vi "Offset Locking- Main with Slave Tracking v2.1.vi"() -> ()   [LabVIEW 2018]
uses:
  <vilib>/Utility/error.llb/DialogType.ctl
  <vilib>/Analysis/1siggen.llb/Ramp Pattern by Samples.vi
  <vilib>/measure/mamon.llb/Waveform Peak Detection for 1 Chan.vi
  <vilib>/addons/control/pid/pid.llb/PID Advanced (DBL).vi
  <vilib>/measure/NI_MAPro.lvlib
  <vilib>/addons/control/pid/NI_PID_pid.lvlib
  <vilib>/Analysis/NI_AALBase.lvlib
  <vilib>/measure/NI_MABase.lvlib
panel:
  in  "width":i32=100
  in  "start":dbl format="%0.2f"
  in  "end":dbl=1.0 format="%0.2f"
  in  "samples":i32=128
  in  "Waveform Test?":bool
  in  "reset signal":bool
  in  "phase":dbl format="%.2p"
  out "Chirp Rate":dbl format="%#_g GHz/ms"
  out "Single Mode?":bool
  out "# of Peaks found when Chirping?":i32
  in  "Minimum amplitude for Slave":dbl=0.15 format="%.2p"
  in  "Minimum \namplitude\nfor peaks":dbl=0.8 format="%#_13g V"
  in  "PZT Voltage to \nFrequency Conversion":dbl=-1.41655 format="%#_g V/GHz"
  out "PZT Chirp Output":waveform(dbl)(graph)
  in  "offset":dbl format="%0.2p V"
  in  "Sampling Info":cluster{"Fs":dbl, "#s":dbl}={"Fs"=10000.0, "#s"=100.0} {"Fs" format="%.2p"}
  in  "frequency":dbl=10.0 format="%0.2p Hz"
  in  "Chirp Amplitude":dbl=1.5 format="%0.2p GHz"
  in  "Run Chirp Program?":bool
  out "Run Time (min)":dbl
  out "standard deviation":dbl format="%0.3e"
  in  "Ref Peak 2":i32=2
  in  "Ref Peak":i32=3
  in  "First Cal Peak":i32=2
  in  "Last Cal Peak":i32=4
  out "# found":i32
  out "Offset":dbl(graph)
  in  "Manual PZT Control":dbl format="%#_g V"
  in  "Engage PZT PID?":bool
  out "Offset (GHz)":dbl format="%#_4g"
  in  "# of Shots for Averaging":i32=100
  in  "Name Convention":string="Chirp Offset Lock Log"
  in  "Save Directory":path=path "C:/Users/LabUser/Google Drive/Measurements/04-2018"
  out "Four peaks?":bool
  out "PZT Output":dbl(graph)
  in  "PID Gains":T1={"proportional gain (Kc)"=-1.0, "integral time (Ti, min)"=0.01, "derivative time (Td, min)"=0.0} {"derivative time (Td, min)" format="%.3f"; "integral time (Ti, min)" format="%.3f"; "proportional gain (Kc)" format="%.3f"}
  in  "Setpoint Range (GHz)":cluster{"setpoint high":dbl, "setpoint low":dbl}={"setpoint high"=7.7901, "setpoint low"=7.7899} {"setpoint high" format="%.4f"; "setpoint low" format="%.4f"}
  out "dt out (s)":dbl format="%.3f"
  in  "Frequency Offset Setpoint (GHz)":dbl=7.79 format="%.3f"
  out "GHz/sec":dbl
  out "dt":dbl format="%#_4g"
  out "Locations":dbl[](array[numeric]) format="%.2p"
  out "Amplitudes":dbl[](array[numeric]) format="%.2p"
  out "2nd Derivatives":dbl[](array[numeric]) format="%.2p"
  out "10 GHz FPI":dynamicdata(graph)
  in  "Stop":bool
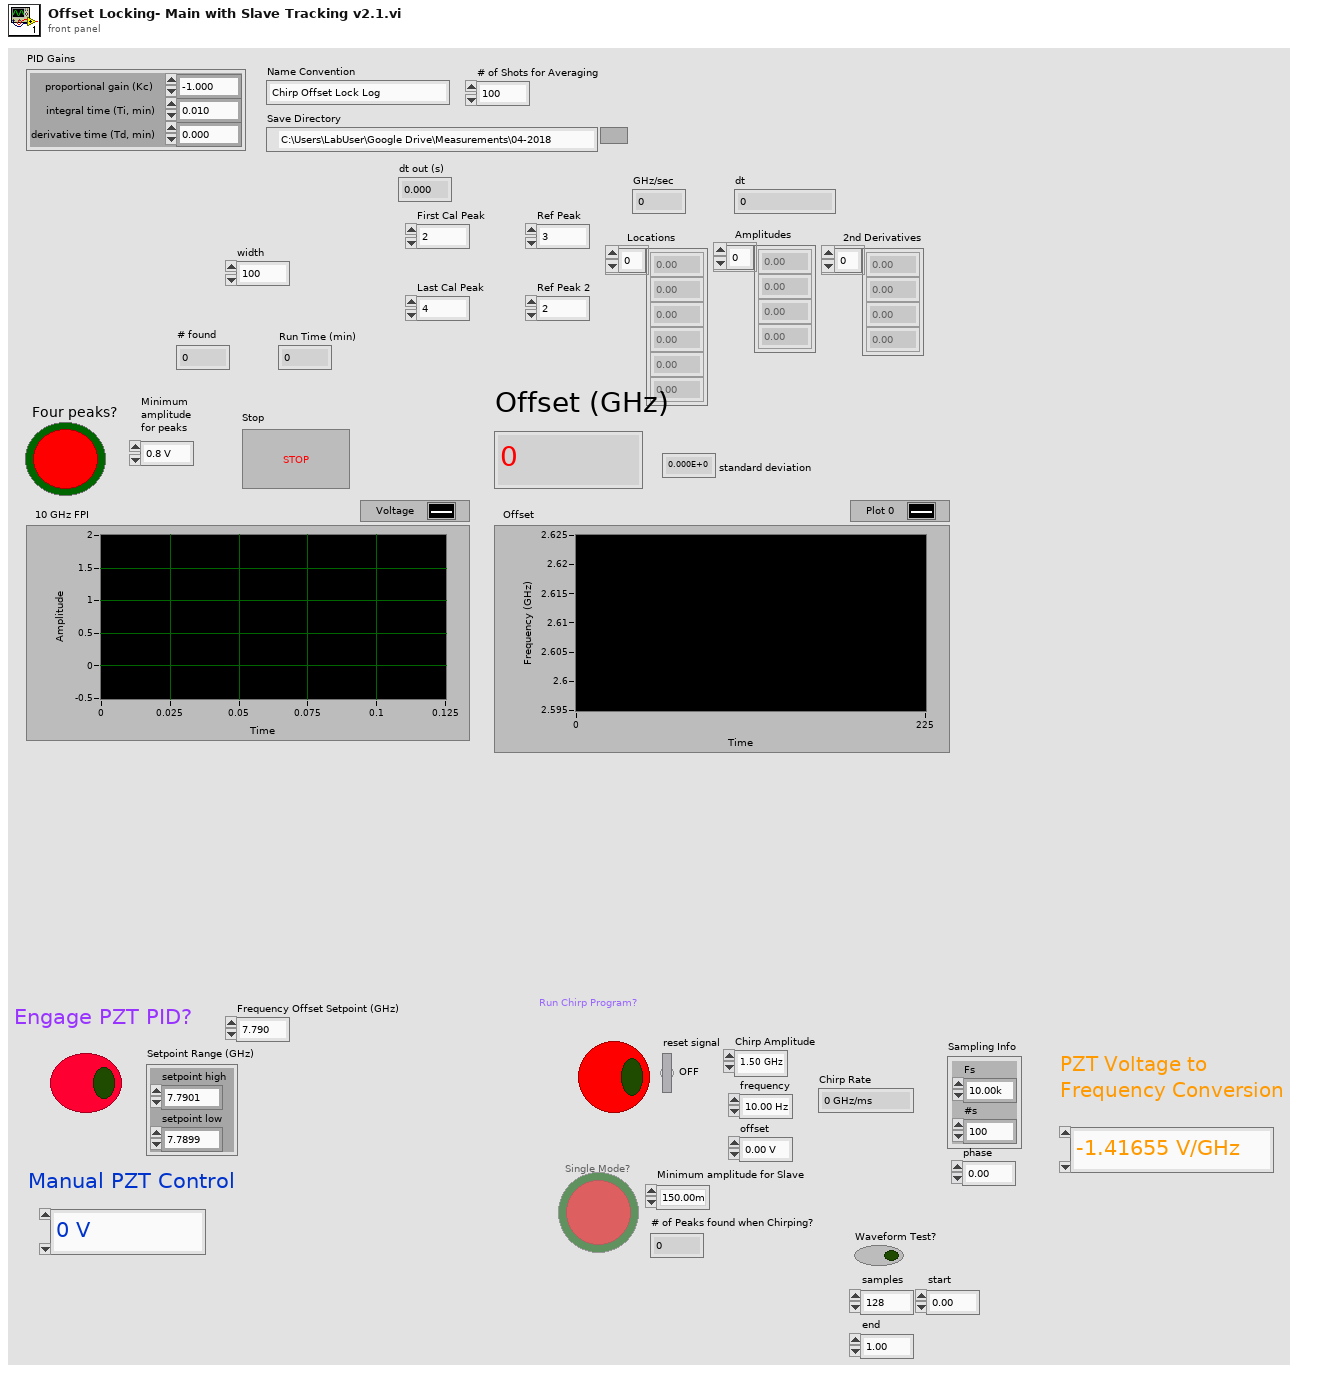
[diagram p1: front panel]
types:
  T1 = cluster{"proportional gain (Kc)":dbl, "integral time (Ti, min)":dbl, "derivative time (Td, min)":dbl}
  T2 = enum8{"Enabled", "Disabled", "Disabled and Grayed Out"}
  T3 = typedef "DialogType.ctl" = u16
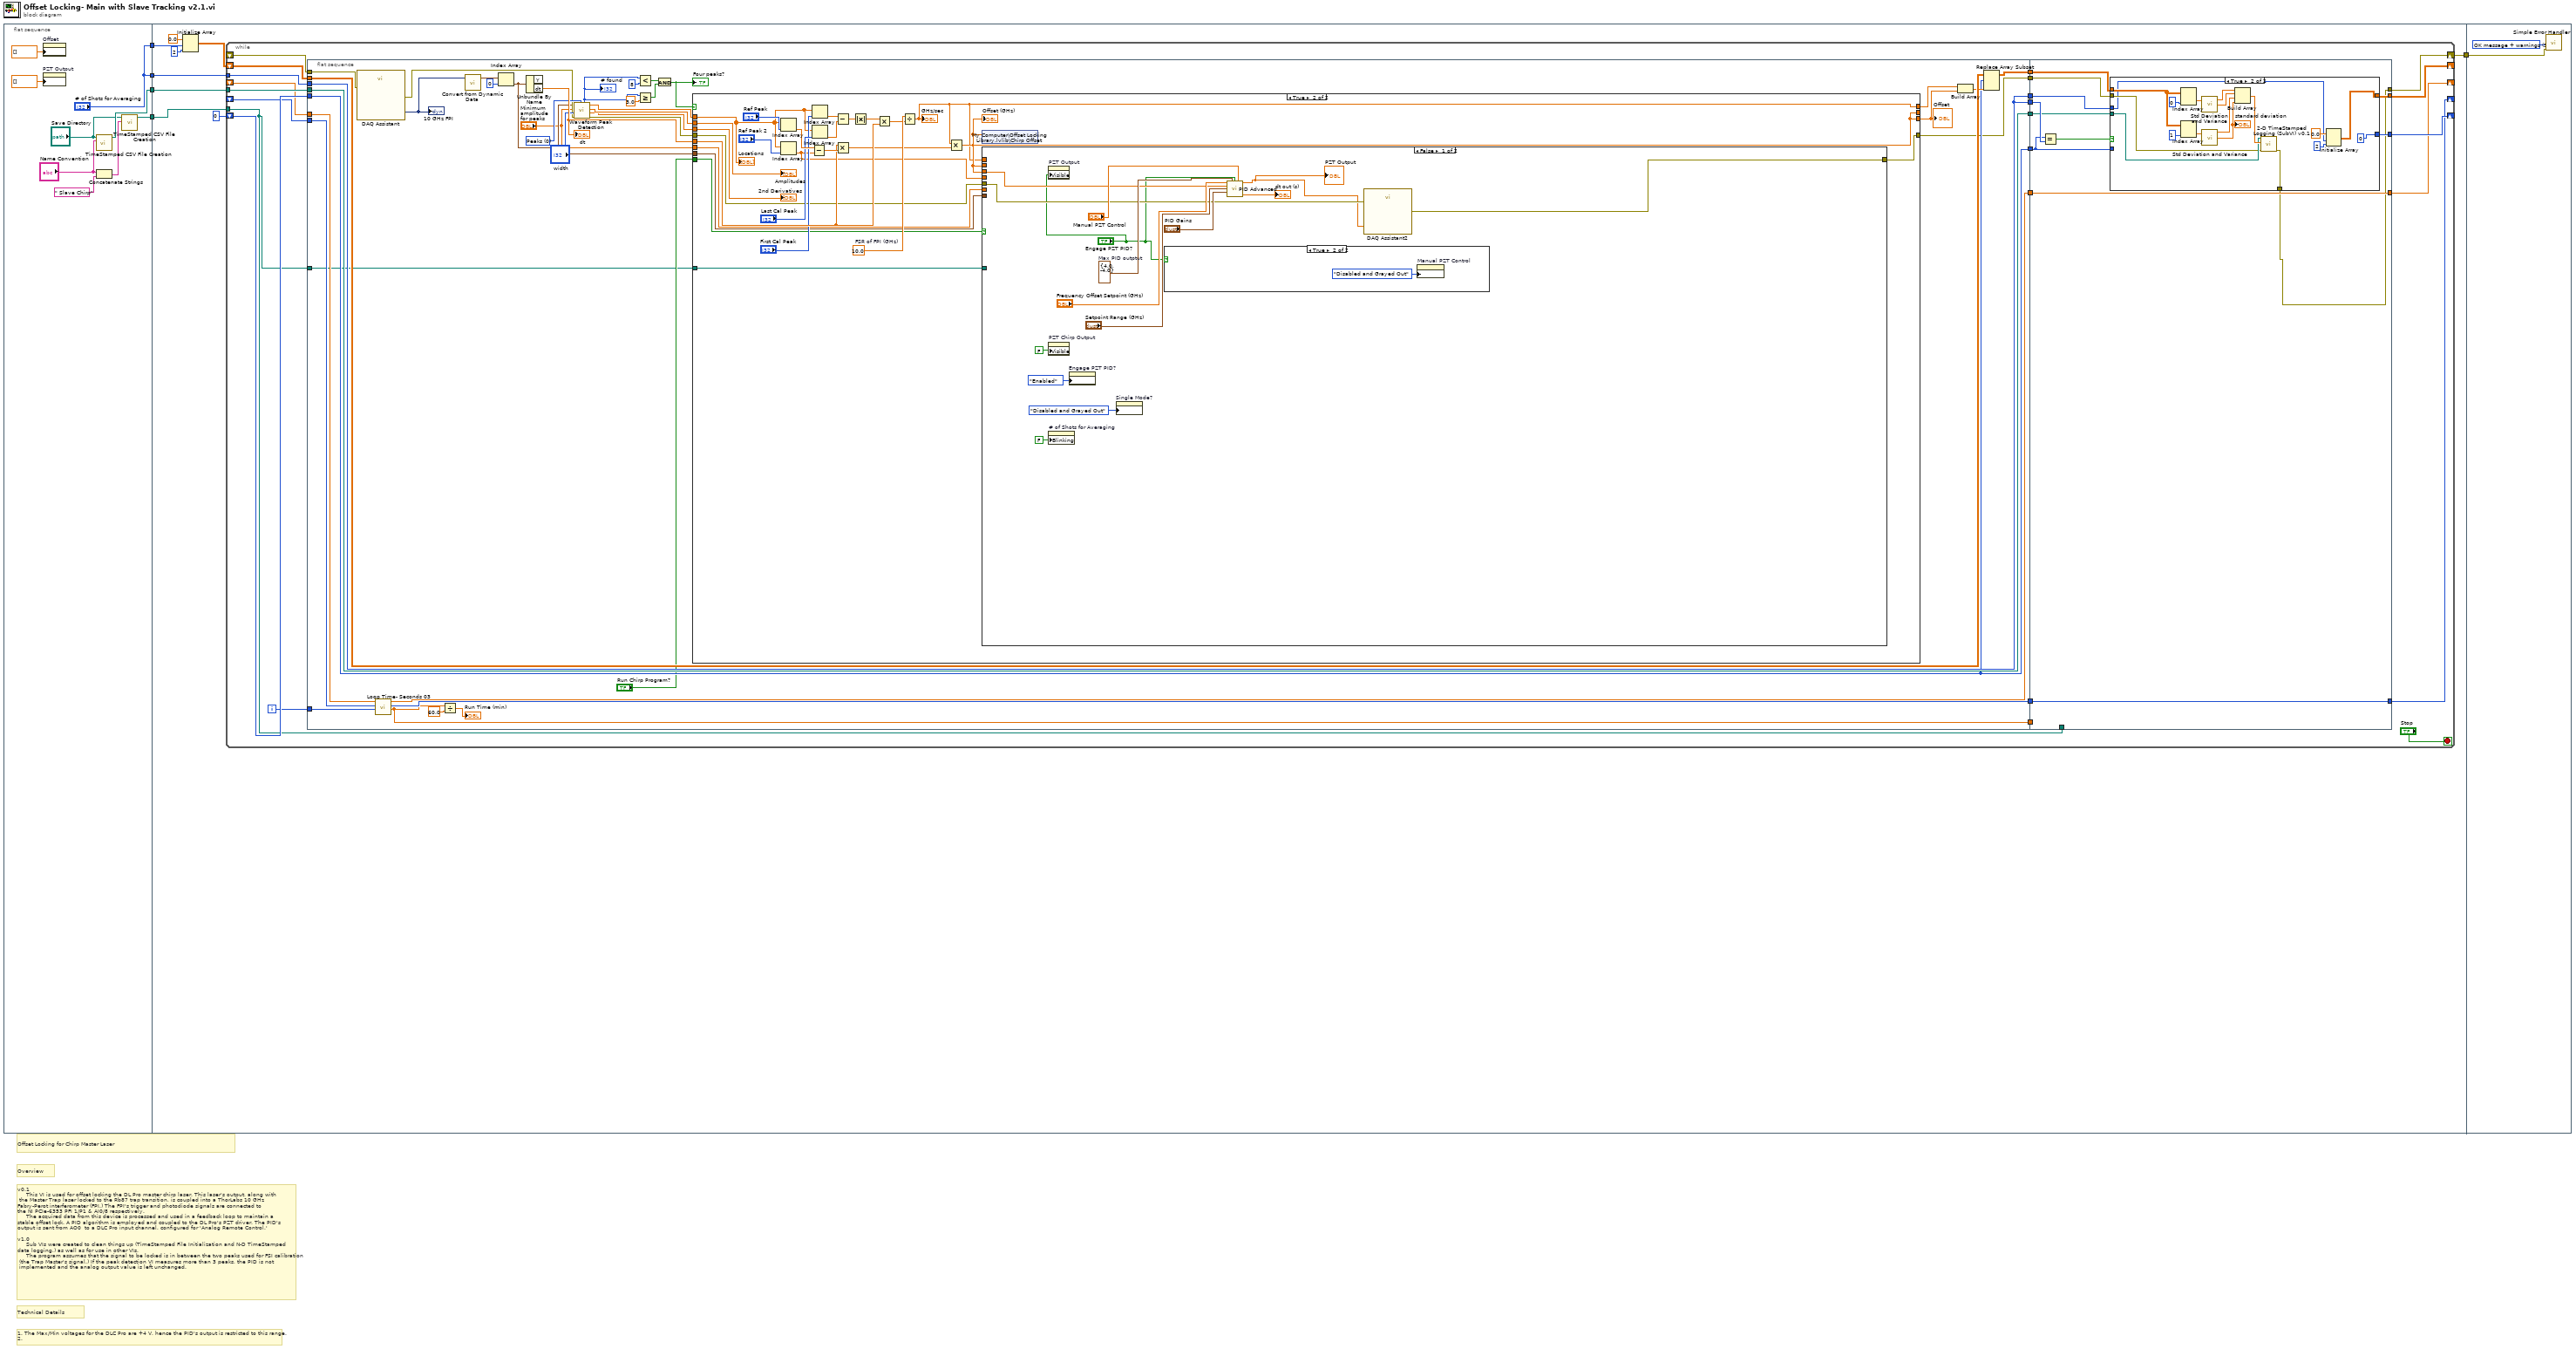
[diagram p0: block diagram]
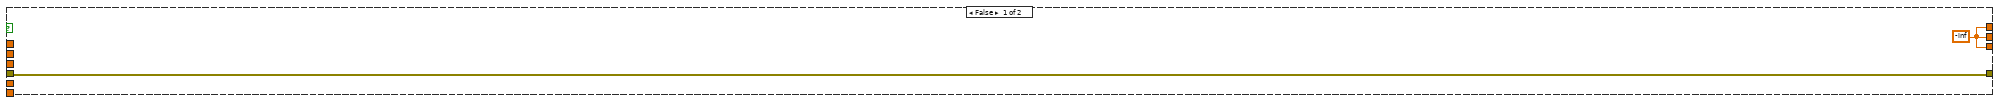
[diagram p2: hidden frame]
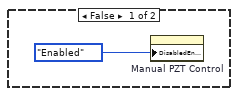
[diagram p3: hidden frame]
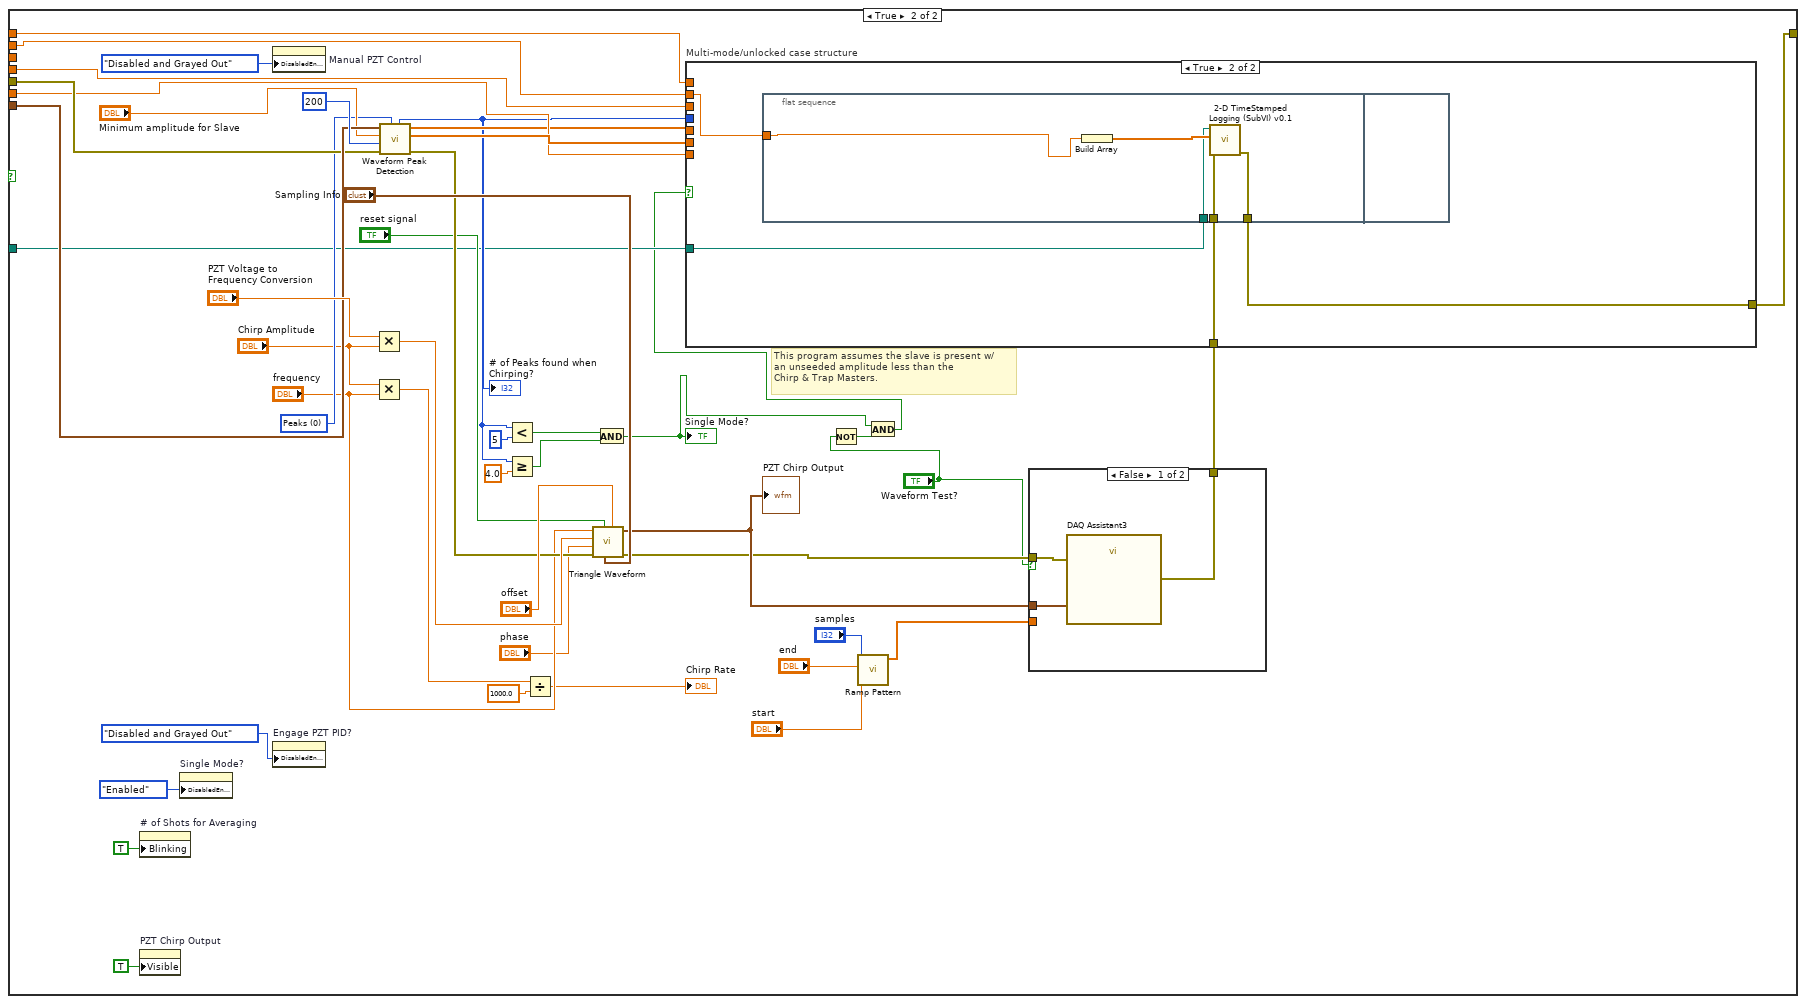
[diagram p4: hidden frame]
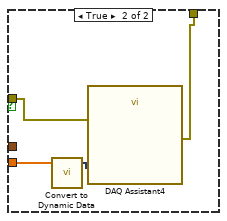
[diagram p5: hidden frame]
diagram:
  # "1. The Max/Min voltages for the DLC Pro are +4 V, hence the PID's output is restricted to this range.\n2."
  # "Technical Details"
  # "v0.1\n     This VI is used for offset locking the DL Pro master chirp laser. This laser's output, along with\n the Master Trap laser locked to the Rb87 trap transition, is coupled into a ThorLabs 10 GHz \nFabry-Perot interferometer (FPI.) The FPI's trigger and photodiode signals are connected to \nthe NI PCIe-6353 PFI 1/P1 & AI0/8 respectively. \n     The acquired data from this device is processed and used in a feedback loop to maintain a \nstable offset lock. A PID algorithm is employed and coupled to the DL Pro's PZT driver. The PID's\noutput is sent from AO0  to a DLC Pro input channel, configured for 'Analog Remote Control.'\n\nv1.0\n     Sub VIs were created to clean things up (TimeStamped File Initialization and N-D TimeStamped \ndata logging,) as well as for use in other VIs.\n     The program assumes that the signal to be locked is in between the two peaks used for FSI calibration\n (the Trap Master's signal.) If the peak detection VI measures more than 3 peaks, the PID is not\n implemented and the analog output value is left unchanged."
  # "Overview"
  # "Offset Locking for Chirp Master Laser"
  n1 = flat-sequence {
    tunnel: [w14] -> w5
    tunnel: ["# of Shots for Averaging"] -> w3
    tunnel: ["# of Shots for Averaging"] -> w2
    tunnel: [w6] -> w1
    tunnel: w5 -> [w23]
    tunnel: [w22] -> w4
    tunnel: w3 -> [w20]
    tunnel: w2 -> [w17]
    tunnel: w1 -> [w15]
    tunnel: w4 -> [w234]
    frame #0 {
      n2 = property on="Offset" class="WFChart (strict)"("History Data"=dbl[] []) -> ()  [unwired: 2 in, 2 out]
      n3 = property on="PZT Output" class="WFChart (strict)"("History Data"=dbl[] []) -> ()  [unwired: 2 in, 2 out]
      n4 = call "TimeStamped CSV File Creation.vi"("Name Convention"="Name Convention", "Save Directory"="Save Directory") -> ("path"=w14:path)  [unwired: 8 in, 1 out]
      n5 = Concatenate Strings("Name Convention", " Slave Chirp" ("string")) -> (w8:string)
      n6 = call "TimeStamped CSV File Creation.vi"("Name Convention"=w8, "Save Directory"="Save Directory") -> ("path"=w6:path)  [unwired: 8 in, 1 out]
    }
    frame #1 {
      n7 = Initialize Array(0.0 ("element"), w17, 2 ("dimension size")) -> (w19:dbl[][])
      n8 = while {
        shift-right: [w35] -> w22
        shift-left: _ -> [w46]
        tunnel: w23 -> [w44]
        shift-right: [w33] -> _
        shift-left: 0 -> [w42]
        tunnel: w20 -> [w40]
        shift-right: [w34] -> _
        shift-left: w19 -> [w37]
        shift-right: [w31] -> _
        shift-left: _ -> [w28]
        shift-right: [w29] -> _
        shift-left: _ -> [w27]
        tunnel: w15 -> [w24]
        i -> [w26]
        stop <- "Stop" stop-if-true
        n9 = flat-sequence {
          tunnel: w46 -> [w76]
          tunnel: [w52] -> w45
          tunnel: w44 -> [w74]
          tunnel: [w74] -> w43
          tunnel: w42 -> [w68]
          tunnel: [w68] -> w41
          tunnel: w40 -> [w69]
          tunnel: [w69] -> w39
          tunnel: [w73] -> w38
          tunnel: w37 -> [w72]
          tunnel: [w69] -> w36
          tunnel: [w67] -> w32
          tunnel: [w66] -> w30
          tunnel: w28 -> [w65]
          tunnel: w27 -> [w64]
          tunnel: w26 -> [w63]
          tunnel: [w55] -> w25
          tunnel: w24 -> [w48]
          tunnel: w45 -> [w207]
          tunnel: w43 -> [w208]
          tunnel: w41 -> [w202]
          tunnel: w39 -> [w212]
          tunnel: w38 -> [w209]
          tunnel: w36 -> [w210]
          tunnel: [w201] -> w35
          tunnel: [w206] -> w34
          tunnel: [w205] -> w33
          tunnel: w32 -> [w204]
          tunnel: [w204] -> w31
          tunnel: [w203] -> w29
          tunnel: w30 -> [w203]
          tunnel: w25 -> [_]
          tunnel: w24 -> [_]
          frame #0 {
            w78 = u16 0 items=["Peaks", "Valleys"] ("peaks/valleys")
            n10 = call "DAQ Assistant"("error in"=w76) -> ("data"=w84:dynamicdata, "error out"=w75:errorcluster)  [unwired: 16 in, 1 out]
            "10 GHz FPI" <- w84
            n11 = call "Loop Time- Seconds 03.vi"("Loop Iteration"=w63, "Shift Registered Time In"=w64, "Shift Registered In"=w65) -> ("t"=w55:dbl, "Shift Registered Time Out"=w66:u32, "Shift Registered Out"=w67:dbl)  [unwired: 6 in]
            n12 = Divide(x=w55, y=60.0) -> (x/y=→"Run Time (min)":dbl)
            n13 = call "Convert from Dynamic Data"("Dynamic Data Type"=w84) -> ("Array of Waveform"=w86:waveform(dbl)[])  [unwired: 3 in]
            n14 = Index Array(array=w86, index=0) -> (element=w50:waveform(dbl))
            n15 = Unbundle By Name(w50) -> ("dt"=w80:dbl)  [unwired: 1 out]
            "dt" <- w80
            n16 = call-poly <vilib>:"Waveform Peak Detection.vi"("peaks/valleys"=w78, "error in"=w75, "width"="width", "threshold"="Minimum \namplitude\nfor peaks", "Signal In"=w50) -> ("error out"=w53:errorcluster, "2nd Derivatives"=w82:dbl[], "Amplitudes"=w83:dbl[], "Locations"=w81:dbl[], "# found"=w60:i32)  [unwired: 2 in]
            "# found" <- w60
            n17 = Less?(x=w60, y=8) -> (x < y?=w58:bool)
            n18 = Greater Or Equal?(x=w60, y=3.0) -> (x >= y?=w61:bool)
            n19 = And(x=w58, y=w61) -> (x .and. y?=w57:bool)
            "Four peaks?" <- w57
            n20 = case shown="True" w57 {
              tunnel: w83 -> [_ w93]
              tunnel: w82 -> [_ w114]
              tunnel: w81 -> [_ w99]
              tunnel: w80 -> [_ w105]
              tunnel: [w88 w90] -> w71
              tunnel: [w88 w94] -> w62
              tunnel: [w88 w94] -> _
              tunnel: w53 -> [w87 w98]
              tunnel: [w87 w97] -> w52
              tunnel: "Run Chirp Program?" -> [_ w96]
              tunnel: w50 -> [_ w95]
              tunnel: "Minimum \namplitude\nfor peaks" -> [_ w92]
              tunnel: w48 -> [_ w89]
              frame False {
                w88 = -inf
              }
              frame True {
                w112 = 10.0  # FSR of FPI (GHz)
                n21 = Index Array(array=w99, index="Ref Peak") -> (element=w107:dbl)
                n22 = Index Array(array=w99, index="Ref Peak 2") -> (element=w91:dbl)
                n23 = Subtract(x=w107, y=w91) -> (x-y=w106:dbl)
                n24 = Index Array(array=w99, index="First Cal Peak") -> (element=w108:dbl)
                n25 = Index Array(array=w99, index="Last Cal Peak") -> (element=w113:dbl)
                n26 = Subtract(x=w108, y=w113) -> (x-y=w110:dbl)
                n27 = Multiply(x=w105, y=w106) -> (x*y=w104:dbl)
                n28 = Absolute Value(x=w110) -> (abs(x)=w109:dbl)
                n29 = Multiply(x=w109, y=w105) -> (x*y=w111:dbl)
                n30 = Divide(x=w112, y=w111) -> (x/y=w90:dbl)
                "GHz/sec" <- w90
                n31 = Multiply(x=w90, y=w104) -> (x*y=w94:dbl)
                "Offset (GHz)" <- w94
                n32 = shared-variable "My Computer\\Offset Locking Library.lvlib\\Chirp Offset"(w94) -> ()  [unwired: 1 in, 1 out]
                n33 = case shown="False" w96 {
                  tunnel: w94 -> [w123 _]
                  tunnel: w98 -> [w122 w167]
                  tunnel: [w121 w140] -> w97
                  tunnel: w95 -> [_ w168]
                  tunnel: w94 -> [_ w164]
                  tunnel: w92 -> [_ w158]
                  tunnel: w91 -> [_ w156]
                  tunnel: w90 -> [_ w155]
                  tunnel: w89 -> [_ w142]
                  frame False {
                    w125 = cluster{"output high":dbl, "output low":dbl} {"output high"=4.0, "output low"=-4.0}  # Max PID outptut
                    n34 = property on="PZT Output" class="WFChart (strict)"("Visible"="Engage PZT PID?") -> ()  [unwired: 2 in, 2 out]
                    n35 = property on="PZT Chirp Output" class="WFGraph (strict)"("Visible"=FALSE) -> ()  [unwired: 2 in, 2 out]
                    n36 = property on="# of Shots for Averaging" class="DigNum (strict)"("Blinking"=FALSE) -> ()  [unwired: 2 in, 2 out]
                    n37 = property on="Engage PZT PID?" class="Bool (strict)"("DisabledEnum"=T2."Enabled" ("Disabled")) -> ()  [unwired: 2 in, 2 out]
                    n38 = property on="Single Mode?" class="Bool (strict)"("DisabledEnum"=T2."Disabled and Grayed Out" ("Disabled")) -> ()  [unwired: 2 in, 2 out]
                    n39 = case shown="True" "Engage PZT PID?" {
                      frame False {
                        n40 = property on="Manual PZT Control" class="DigNum (strict)"("DisabledEnum"=T2."Enabled" ("Disabled")) -> ()  [unwired: 2 in, 2 out]
                      }
                      frame True {
                        n41 = property on="Manual PZT Control" class="DigNum (strict)"("DisabledEnum"=T2."Disabled and Grayed Out" ("Disabled")) -> ()  [unwired: 2 in, 2 out]
                      }
                    }
                    n42 = call-poly <vilib>:"PID Advanced.vi"("setpoint"="Frequency Offset Setpoint (GHz)", "output range"=w125, "auto? (T)"="Engage PZT PID?", "manual control"="Manual PZT Control", "process variable"=w123, "setpoint range"="Setpoint Range (GHz)", "PID gains"="PID Gains") -> ("output"=w120:dbl, "dt out (s)"=→"dt out (s)":dbl)  [unwired: 7 in]
                    "PZT Output" <- w120
                    n43 = call "DAQ Assistant2"("data"=w120, "error in"=w122) -> ("error out"=w121:errorcluster)  [unwired: 16 in, 1 out]
                  }
                  frame True {
                    w154 = u16 0 items=["Peaks", "Valleys"] ("peaks/valleys")
                    # "This program assumes the slave is present w/ \nan unseeded amplitude less than the \nChirp & Trap Masters."
                    n44 = property on="# of Shots for Averaging" class="DigNum (strict)"("Blinking"=TRUE) -> ()  [unwired: 2 in, 2 out]
                    n45 = property on="PZT Chirp Output" class="WFGraph (strict)"("Visible"=TRUE) -> ()  [unwired: 2 in, 2 out]
                    n46 = property on="Single Mode?" class="Bool (strict)"("DisabledEnum"=T2."Enabled" ("Disabled")) -> ()  [unwired: 2 in, 2 out]
                    n47 = property on="Manual PZT Control" class="DigNum (strict)"("DisabledEnum"=T2."Disabled and Grayed Out" ("Disabled")) -> ()  [unwired: 2 in, 2 out]
                    n48 = property on="Engage PZT PID?" class="Bool (strict)"("DisabledEnum"=T2."Disabled and Grayed Out" ("Disabled")) -> ()  [unwired: 2 in, 2 out]
                    n49 = Multiply(x="PZT Voltage to \nFrequency Conversion", y="Chirp Amplitude") -> (x*y=w170:dbl)
                    n50 = Multiply(x="Chirp Amplitude", y="frequency") -> (x*y=w149:dbl)
                    n51 = call-poly <vilib>:"Waveform Peak Detection.vi"("peaks/valleys"=w154, "error in"=w167, "width"=200, "threshold"="Minimum amplitude for Slave", "Signal In"=w168) -> ("error out"=w166:errorcluster, "Amplitudes"=w159:dbl[], "Locations"=w157:dbl[], "# found"=w143:i32)  [unwired: 2 in, 1 out]
                    "# of Peaks found when Chirping?" <- w143
                    n52 = Less?(x=w143, y=5) -> (x < y?=w160:bool)
                    n53 = Greater Or Equal?(x=w143, y=4.0) -> (x >= y?=w162:bool)
                    n54 = Divide(x=w149, y=1000.0) -> (x/y=→"Chirp Rate":dbl)
                    n55 = call <vilib>:"Triangle Waveform.vi"("offset"="offset", "sampling info"="Sampling Info", "reset signal"="reset signal", "error in (no error)"=w166, "phase"="phase", "amplitude"=w170, "frequency"="frequency") -> ("error out"=w144:errorcluster, "signal out"=w145:waveform(dbl))  [unwired: 3 in]
                    "PZT Chirp Output" <- w145
                    n56 = And(x=w160, y=w162) -> (x .and. y?=w138:bool)
                    "Single Mode?" <- w138
                    n57 = Not(x="Waveform Test?") -> (.not. x?=w139:bool)
                    n58 = call-poly <vilib>:"Ramp Pattern.vi"("start"="start", "end"="end", "samples"="samples") -> ("Ramp Pattern"=w135:dbl[])  [unwired: 7 in, 1 out]
                    n59 = And(x=w138, y=w139) -> (x .and. y?=w137:bool)
                    n60 = case shown="False" "Waveform Test?" {
                      tunnel: w145 -> [w180 _]
                      tunnel: w144 -> [w179 w184]
                      tunnel: [w178 w183] -> w141
                      tunnel: w135 -> [_ w182]
                      frame False {
                        n61 = call "DAQ Assistant3"("data"=w180, "error in"=w179) -> ("error out"=w178:errorcluster)  [unwired: 16 in, 1 out]
                      }
                      frame True {
                        n62 = call "Convert to Dynamic Data"("Array"=w182) -> ("Dynamic Data Type"=w181:dynamicdata)  [unwired: 3 in]
                        n63 = call "DAQ Assistant4"("data"=w181, "error in"=w184) -> ("error out"=w183:errorcluster)  [unwired: 16 in, 1 out]
                      }
                    }
                    n64 = case "Multi-mode/unlocked case structure" shown="True" w137 {
                      tunnel: w164 -> [_ w195]
                      tunnel: w143 -> [w191 _]
                      tunnel: w159 -> [w190 _]
                      tunnel: w158 -> [w189 _]
                      tunnel: w157 -> [w188 _]
                      tunnel: w156 -> [w187 _]
                      tunnel: w155 -> [w186 _]
                      tunnel: w142 -> [_ w194]
                      tunnel: w141 -> [w185 w193]
                      tunnel: [w185 w192] -> w140
                      frame False {
                        n65 = for {
                          N: w191 -> [_]
                          tunnel: w190 -> [_] mode=indexing
                          tunnel: w189 -> [_]
                          tunnel: w188 -> [_] mode=indexing
                          tunnel: w187 -> [_]
                          tunnel: w186 -> [_]
                        }
                      }
                      frame True {
                        n66 = flat-sequence {
                          tunnel: w195 -> [w200]
                          tunnel: w194 -> [w198]
                          tunnel: w193 -> [w197]
                          tunnel: [w196] -> w192
                          frame #0 {
                            n67 = Build Array(w200) -> (w199:dbl[])
                            n68 = call "2-D TimeStamped Logging (SubVI) v0.1.vi"("error in (no error)"=w197, "array"=w199, "path"=w198) -> ("error out"=w196:errorcluster)  [unwired: 8 in]
                          }
                          frame #1 {
                          }
                        }
                      }
                    }
                  }
                }
                "2nd Derivatives" <- w114
                "Amplitudes" <- w93
                "Locations" <- w99
              }
            }
            "Offset" <- w62
            n69 = Build Array(w71, w62) -> (w70:dbl[])
            n70 = Replace Array Subset(array=w72, new element=w70, index (row)=w68) -> (w73:dbl[][])  [unwired: 1 in]
          }
          frame #1 {
            n71 = Equal?(x=w202, y=w212) -> (x = y?=w211:bool)
            n72 = case shown="True" w211 {
              tunnel: w210 -> [_ w216]
              tunnel: w209 -> [w215 w229]
              tunnel: w208 -> [_ w223]
              tunnel: w207 -> [w213 w222]
              tunnel: [w215 w219] -> w206
              tunnel: w202 -> [w214 _]
              tunnel: [w214 0] -> w205
              tunnel: [w213 w217] -> w201
              frame False {
              }
              frame True {
                n73 = Index Array(array=w229, index (col)=0 ("disabled index (col)")) -> (element=w232:dbl[])  [unwired: 1 in]
                n74 = Index Array(array=w229, index (col)=1 ("disabled index (col)")) -> (element=w230:dbl[])  [unwired: 1 in]
                n75 = call <vilib>:"Std Deviation and Variance.vi"("X"=w232) -> ("mean"=w228:dbl, "standard deviation"=w227:dbl)  [unwired: 1 in, 1 out]
                n76 = call <vilib>:"Std Deviation and Variance.vi"("X"=w230) -> ("mean"=w226:dbl, "standard deviation"=w225:dbl)  [unwired: 1 in, 1 out]
                "standard deviation" <- w225
                n77 = Build Array(w228, w227, w226, w225) -> (w224:dbl[])
                n78 = call "2-D TimeStamped Logging (SubVI) v0.1.vi"("error in (no error)"=w222, "array"=w224, "path"=w223) -> ("error out"=w217:errorcluster)  [unwired: 8 in]
                n79 = Initialize Array(0.0 ("element"), w216, 2 ("dimension size")) -> (w219:dbl[][])
              }
            }
          }
        }
      }
    }
    frame #2 {
      w235 = T3 3 items=["no dialog", "OK message", "continue or stop message", "OK message + warnings", "continue/stop + warnings"] ("type of dialog (OK msg:1)")
      n80 = call <vilib>:"Simple Error Handler.vi"("type of dialog (OK msg:1)"=w235, "error in (no error)"=w234) -> ()  [unwired: 3 in, 5 out]
    }
  }
